vi "数据库配置.vi"() -> ()   [LabVIEW 2020]
uses:
  <vilib>/Utility/miscctls.llb/LVStringsAndValuesArrayTypeDef_U16.ctl
  <vilib>/addons/database/Connection.llb/DB Tools Open Connec (String).vi
  <vilib>/addons/database/Connection.llb/Conn Execute.vi
  <vilib>/addons/database/Recordset.llb/Rec Fetch Recordset Data (R).vi
  <vilib>/addons/database/Recordset.llb/Rec Destroy - Connection.vi
  <vilib>/addons/database/NI_Database_API.lvlib
panel:
  in  "取消":bool
  in  "确定":bool
  in  "数据库选择":enum32{"单机", "联机追溯"}(tab)
  out "数据库名称（单机）":string
  in  "使用文件名（单机）":string
  in  "打开路径（单机）":bool
  in  "数据库路径（单机）":string
  out "附加数据库（单机）":bool
  out "选择数据库（单机）":bool
  in  "在服务器上选择数据库（单机）":u16(ring) items=["CEPS", "D:\\LOCALDB.MDF", "SANLIserver"]
  in  "测试数据库（单机）":bool
  out "数据库信息":string
  in  "测试数据库（服务器）":bool
  in  "密码":string
  in  "用户名称":string
  in  "服务器名称（服务器）":string
  out "选择数据库（服务器）":bool
  in  "在服务器上选择数据库（服务器）":u16(ring)
  in  "使用文件名（服务器）":string
  in  "打开路径（服务器）":bool
  in  "数据库路径（服务器）":string
  out "附加数据库（服务器）":bool
  # "数据库名称"
  # "使用文件名"
  # "数据库信息"
  # "请输入登陆服务器信息："
  # "使用文件名"
  # "密码"
  # "用户名称"
  # "请输入服务器名称："
  # "服务器名称"
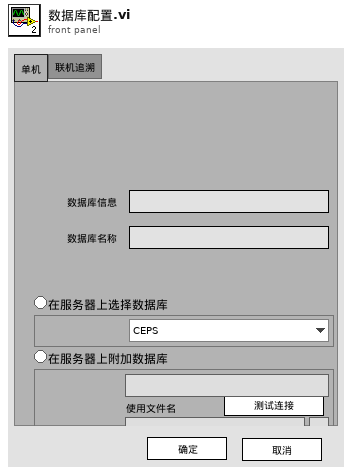
[diagram p1: front panel]
types:
  T1 = typedef "LVStringsAndValuesArrayTypeDef_U16.ctl" = cluster{"String":string, "Value":u16}[]
  T2 = enum8{"Enabled", "Disabled", "Disabled and Grayed Out"}
  T3 = typedef "NI_Database_API.lvlib/Conn ObjectReference.ctl" = refnum<k1>
  T4 = typedef "NI_Database_API.lvlib/Rec ObjectReference.ctl" = refnum<k1>
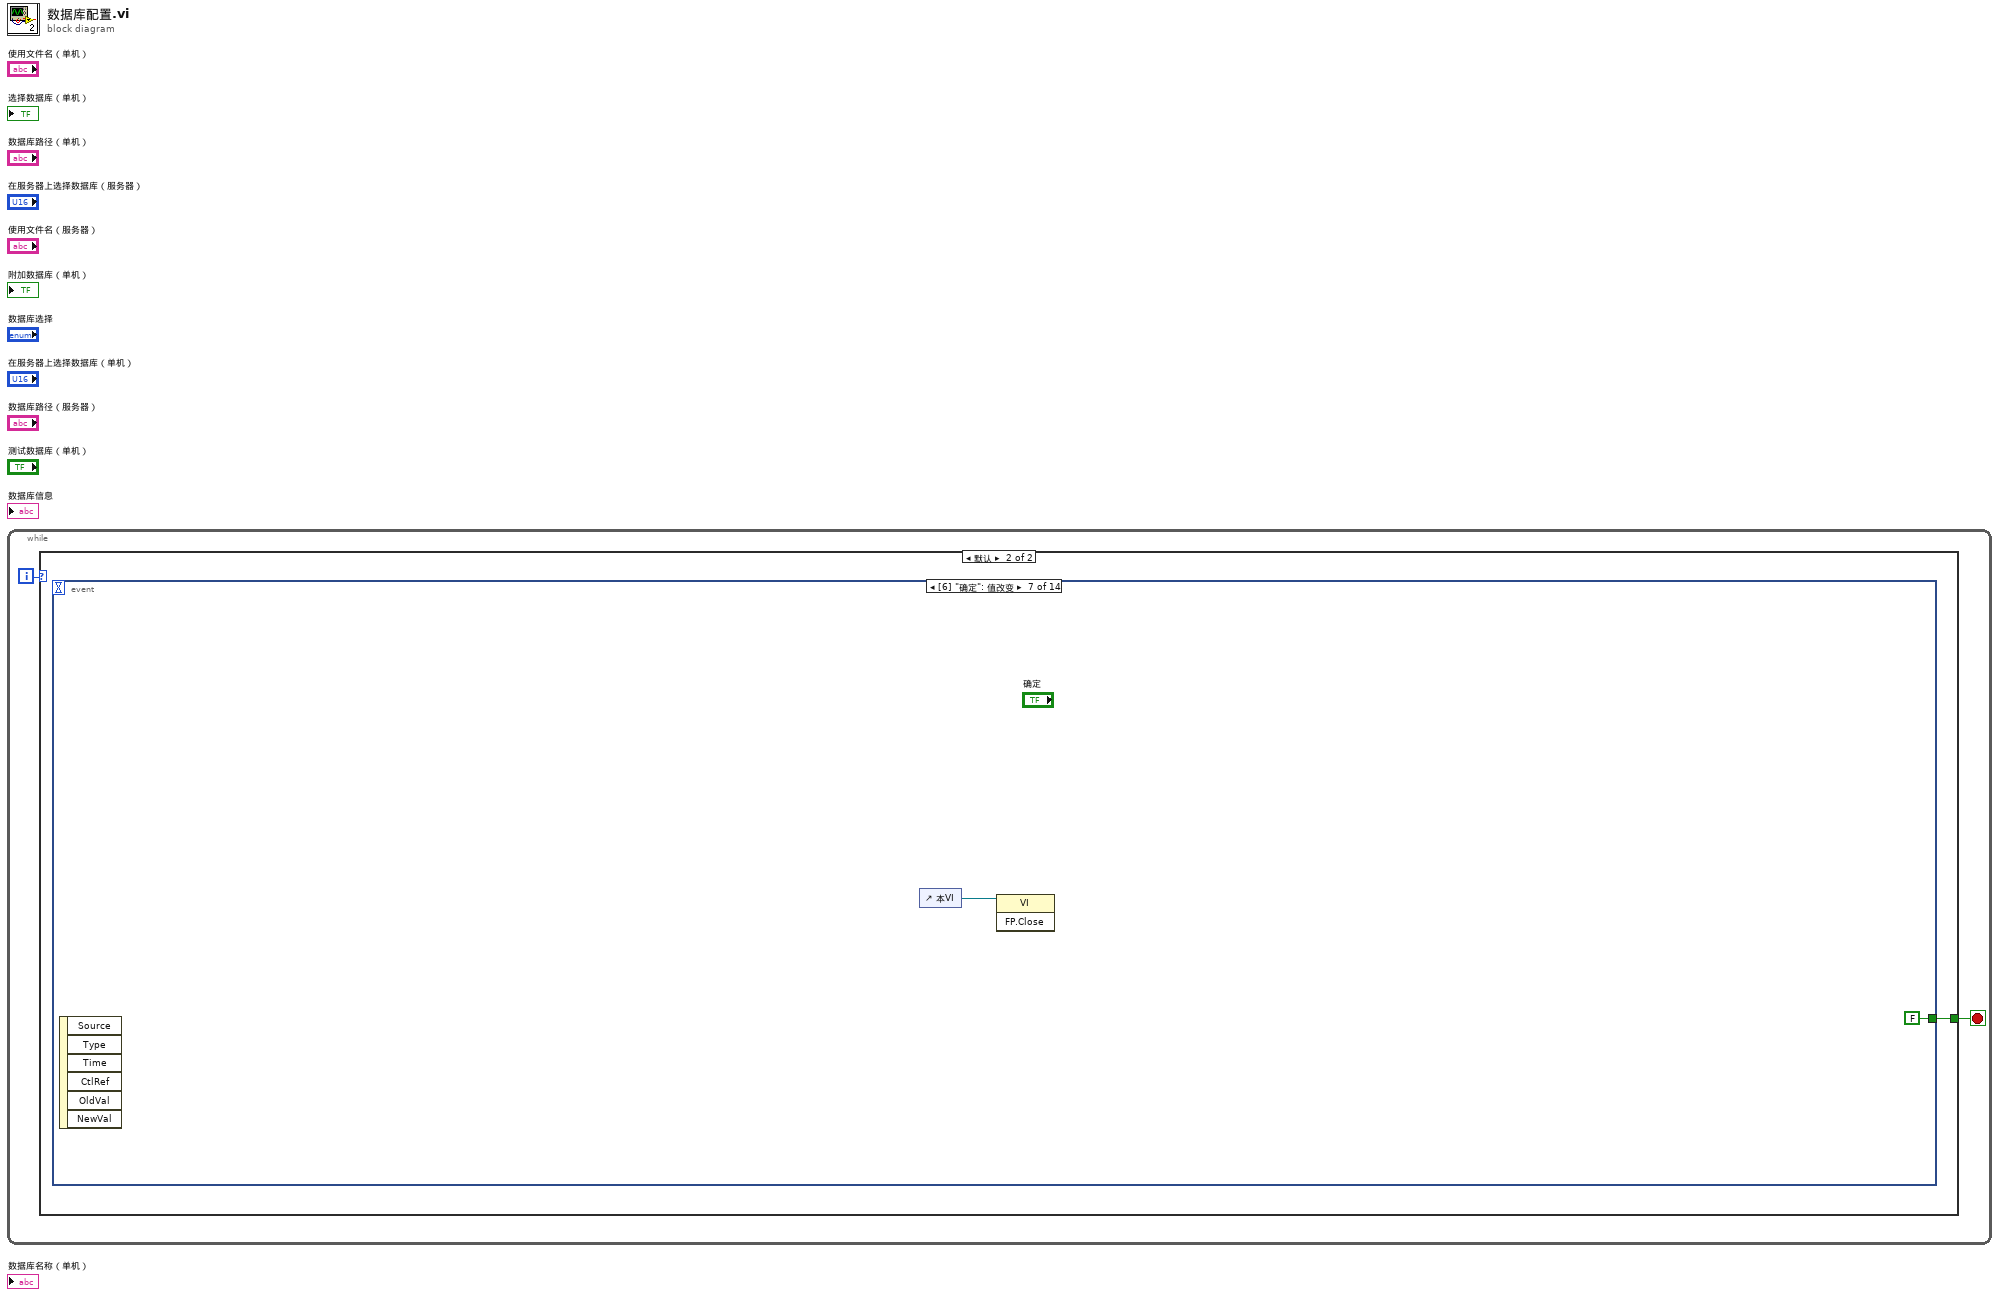
[diagram p0: block diagram]
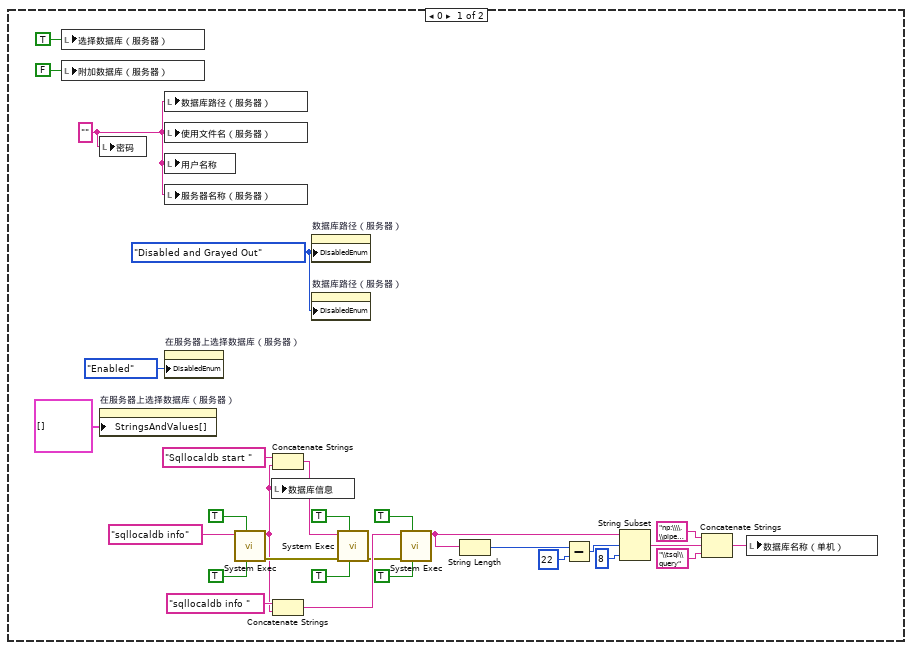
[diagram p2: hidden frame]
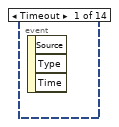
[diagram p3: hidden frame]
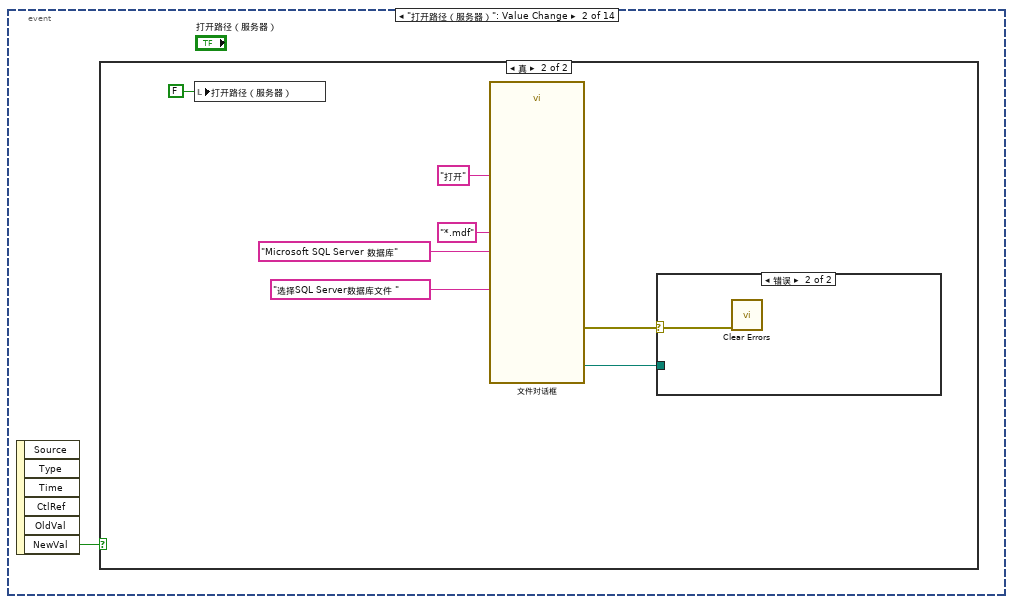
[diagram p4: hidden frame]
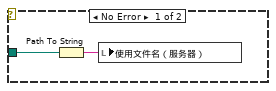
[diagram p6: hidden frame]
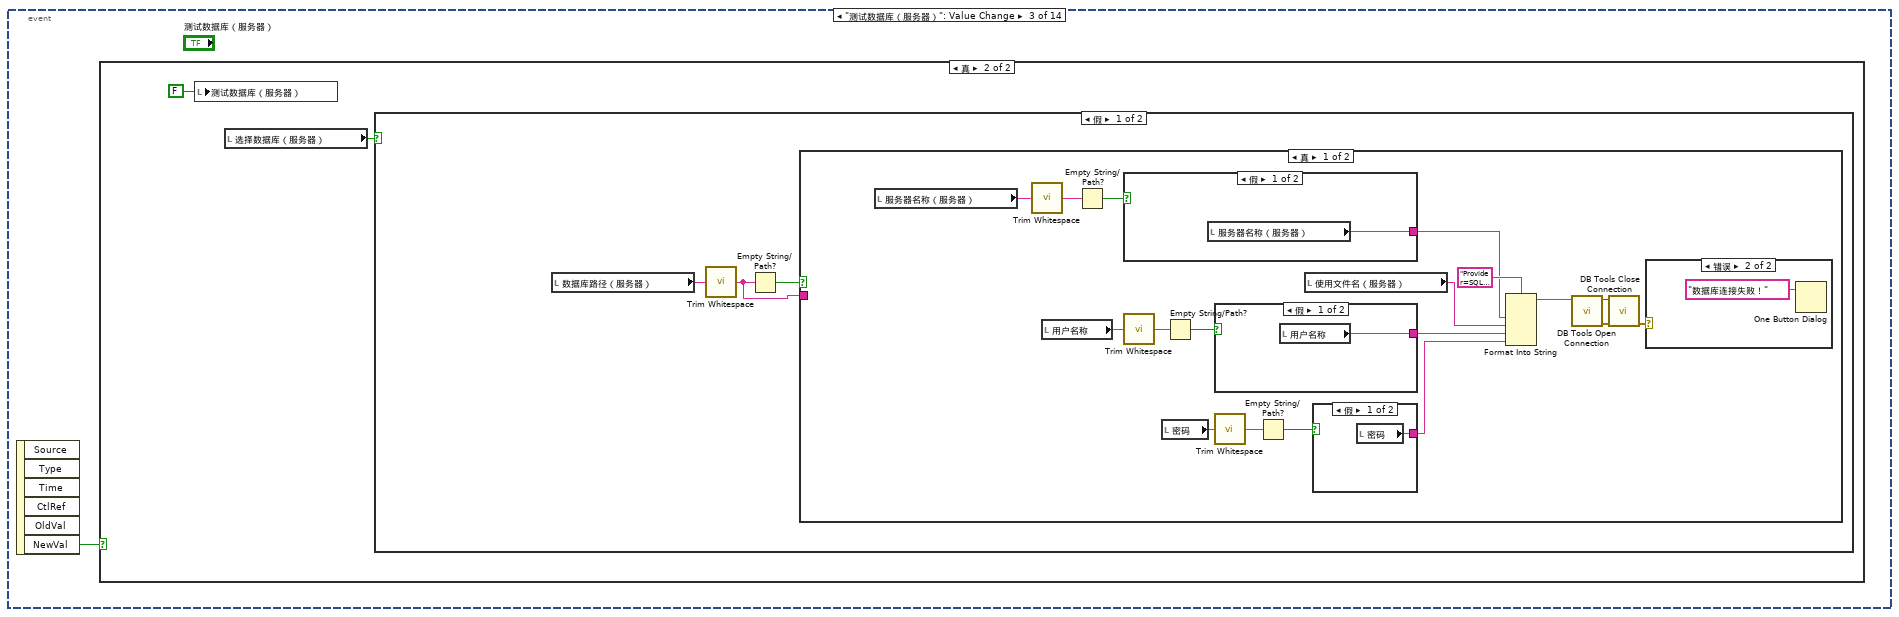
[diagram p7: hidden frame]
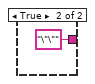
[diagram p9: hidden frame]
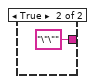
[diagram p10: hidden frame]
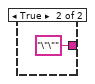
[diagram p11: hidden frame]
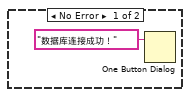
[diagram p12: hidden frame]
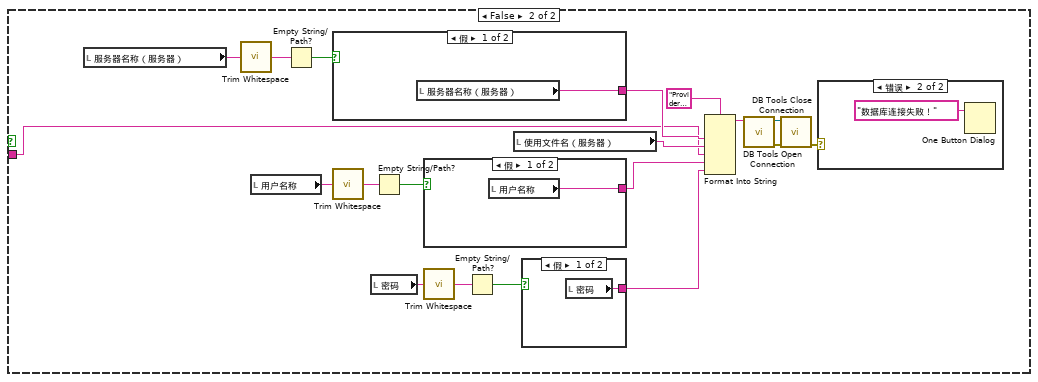
[diagram p13: hidden frame]
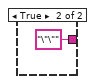
[diagram p14: hidden frame]
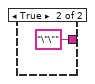
[diagram p15: hidden frame]
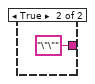
[diagram p16: hidden frame]
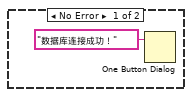
[diagram p17: hidden frame]
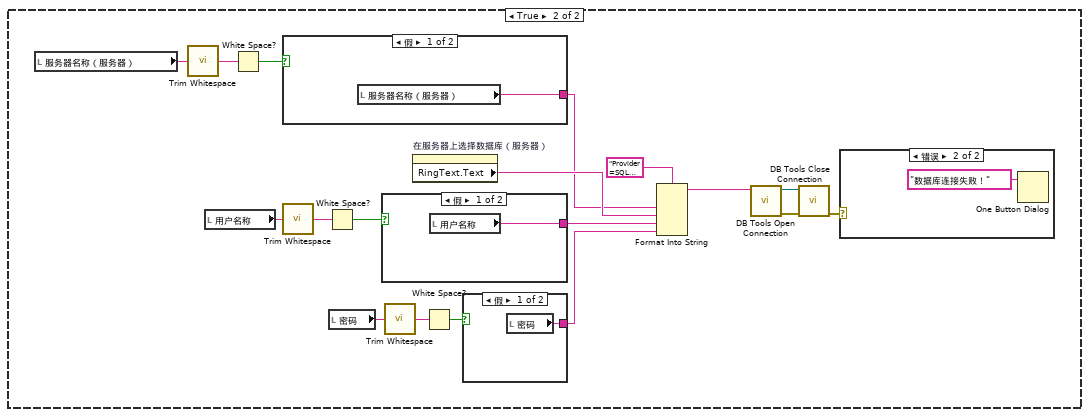
[diagram p18: hidden frame]
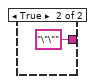
[diagram p19: hidden frame]
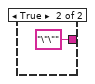
[diagram p20: hidden frame]
diagram:
  n1 = while {
    i -> [w1]
    stop <- w2 stop-if-true
    n2 = case shown="默认" w1 {
      tunnel: [_ w32] -> w2
      frame 0 {
        w27 = ""
        w31 = T2."Disabled and Grayed Out" ("禁用")
        n3 = local write "选择数据库（服务器）"(TRUE ("选择数据库（服务器）")) -> ()
        n4 = local write "附加数据库（服务器）"(FALSE ("附加数据库（服务器）")) -> ()
        n5 = local write "密码"(w27) -> ()
        n6 = property on="在服务器上选择数据库（服务器）" class="Ring (严格)"("StringsAndValues[]"=T1 [] ("字符串与值[]")) -> ()  [unwired: 2 in, 2 out]
        n7 = local write "数据库路径（服务器）"(w27) -> ()
        n8 = local write "使用文件名（服务器）"(w27) -> ()
        n9 = local write "用户名称"(w27) -> ()
        n10 = local write "服务器名称（服务器）"(w27) -> ()
        n11 = property on="在服务器上选择数据库（服务器）" class="Ring (严格)"("DisabledEnum"=T2."Enabled" ("禁用")) -> ()  [unwired: 2 in, 2 out]
        n12 = call <vilib>:"System Exec.vi"("run minimized? (F)"=TRUE, "wait until completion? (T)"=TRUE, "command line"="sqllocaldb info") -> ("error out"=w18:errorcluster, "standard output"=w5:string)  [unwired: 5 in, 2 out]
        n13 = local write "数据库信息"(w5) -> ()
        n14 = Concatenate Strings("Sqllocaldb start " ("command line"), w5) -> (w19:string)
        n15 = Concatenate Strings("sqllocaldb info " ("command line"), w5) -> (w17:string)
        n16 = property on="数据库路径（服务器）" class="Str"("DisabledEnum"=w31) -> ()  [unwired: 2 in, 2 out]
        n17 = property on="数据库路径（服务器）" class="Str"("DisabledEnum"=w31) -> ()  [unwired: 2 in, 2 out]
        n18 = call <vilib>:"System Exec.vi"("run minimized? (F)"=TRUE, "wait until completion? (T)"=TRUE, "error in (no error)"=w18, "command line"=w19) -> ("error out"=w4:errorcluster)  [unwired: 4 in, 3 out]
        n19 = call <vilib>:"System Exec.vi"("run minimized? (F)"=TRUE, "wait until completion? (T)"=TRUE, "error in (no error)"=w4, "command line"=w17) -> ("standard output"=w12:string)  [unwired: 4 in, 3 out]
        n20 = String Length(string=w12) -> (length=w13:i32)
        n21 = Subtract(x=w13, y=22) -> (x-y=w15:i32)
        n22 = String Subset(string=w12, offset (0)=w15, length (rest)=8 ("长度（剩余）")) -> (substring=w8:string)
        n23 = Concatenate Strings("np:\\\\.\\pipe\\LOCALDB#" ("格式字符串"), w8, "\\tsql\\query" ("字符串")) -> (w3:string)
        n24 = local write "数据库名称（单机）"(w3) -> ()
      }
      frame Default {
        n25 = event shown="[6] \"确定\": 值改变" {
          selector: _ -> [_ _ _ _ _ _ _ _ _ _ _ _ _ _]
          dyn-events: _ -> [_ _ _ _ _ _ _ _ _ _ _ _ _ _]
          timeout: _ -> [_ _ _ _ _ _ _ _ _ _ _ _ _ _]
          tunnel: [_ _ _ _ _ _ FALSE TRUE _ _ _ _ _ TRUE] -> w32
          event Timeout {
            n26 = event-data() -> ()  [unwired: 1 in, 3 out]
          }
          event "打开路径（服务器）": Value Change {
            n27 = event-data() -> ("NewVal"=w33:bool)  [unwired: 1 in, 5 out]
            n28 = case shown="真" w33 {
              frame False {
              }
              frame True {
                n29 = local write "打开路径（服务器）"(FALSE ("打开路径（服务器）")) -> ()
                n30 = call "文件对话框"("prompt"="选择SQL Server数据库文件 ", "button label"="打开", "pattern (all files)"="*.mdf", "pattern label"="Microsoft SQL Server 数据库") -> ("selected path"=w36:path, "error out"=w35:errorcluster)  [unwired: 8 in, 2 out]
                n31 = case shown="错误" w35 {
                  selector: w35 -> [_ w43]
                  tunnel: w36 -> [w42 _]
                  frame No Error {
                    n32 = Path To String(path=w42) -> (string=w41:string)
                    n33 = local write "使用文件名（服务器）"(w41) -> ()
                  }
                  frame Error {
                    n34 = call <vilib>:"Clear Errors.vi"("error in (no error)"=w43) -> ()  [unwired: 5 in, 2 out]
                  }
                }
              }
            }
          }
          event "测试数据库（服务器）": Value Change {
            n35 = event-data() -> ("NewVal"=w44:bool)  [unwired: 1 in, 5 out]
            n36 = case shown="真" w44 {
              frame False {
              }
              frame True {
                n37 = local write "测试数据库（服务器）"(FALSE ("测试数据库（服务器）")) -> ()
                n38 = local read "选择数据库（服务器）"() -> (w45:bool)
                n39 = case shown="假" w45 {
                  frame False {
                    n40 = local read "数据库路径（服务器）"() -> (w49:string)
                    n41 = call <vilib>:"Trim Whitespace.vi"("string"=w49) -> ("trimmed string"=w47:string)  [unwired: 1 in]
                    n42 = Empty String/Path?(string/path=w47) -> (empty?=w48:bool)
                    n43 = case shown="真" w48 {
                      tunnel: w47 -> [_ w76]
                      frame True {
                        n44 = local read "服务器名称（服务器）"() -> (w62:string)
                        n45 = call <vilib>:"Trim Whitespace.vi"("string"=w62) -> ("trimmed string"=w60:string)  [unwired: 1 in]
                        n46 = local read "用户名称"() -> (w57:string)
                        n47 = Empty String/Path?(string/path=w60) -> (empty?=w61:bool)
                        n48 = case shown="假" w61 {
                          tunnel: [w72 "\"\""] -> w59
                          frame False {
                            n49 = local read "服务器名称（服务器）"() -> (w72:string)
                          }
                          frame True {
                          }
                        }
                        n50 = call <vilib>:"Trim Whitespace.vi"("string"=w57) -> ("trimmed string"=w53:string)  [unwired: 1 in]
                        n51 = local read "密码"() -> (w58:string)
                        n52 = Empty String/Path?(string/path=w53) -> (empty?=w54:bool)
                        n53 = case shown="假" w54 {
                          tunnel: [w70 "\"\""] -> w52
                          frame False {
                            n54 = local read "用户名称"() -> (w70:string)
                          }
                          frame True {
                          }
                        }
                        n55 = call <vilib>:"Trim Whitespace.vi"("string"=w58) -> ("trimmed string"=w55:string)  [unwired: 1 in]
                        n56 = Empty String/Path?(string/path=w55) -> (empty?=w56:bool)
                        n57 = local read "使用文件名（服务器）"() -> (w50:string)
                        n58 = case shown="假" w56 {
                          tunnel: [w68 "\"\""] -> w51
                          frame False {
                            n59 = local read "密码"() -> (w68:string)
                          }
                          frame True {
                          }
                        }
                        n60 = Format Into String(format string="Provider=SQLOLEDB.1;Integrated Security=SSPI;Persist Security Info=True;Data Source=%s;Initial File Name=%s;User ID=%s;Password=%s" ("格式字符串"), w59, w50, w52, w51) -> (resulting string=w65:string)  [unwired: 2 in, 1 out]
                        n61 = call-poly <vilib>:"DB Tools Open Connection.vi"("connection information"=w65) -> ("error out"=w66:errorcluster, "connection reference"=w67:T3)  [unwired: 7 in]
                        n62 = call <vilib>:"DB Tools Close Connection.vi"("error in (no error)"=w66, "connection reference"=w67) -> ("error out"=w64:errorcluster)  [unwired: 5 in]
                        n63 = case shown="错误" w64 {
                          frame No Error {
                            n64 = One Button Dialog(message="数据库连接成功！" ("消息")) -> ()  [unwired: 1 in, 1 out]
                          }
                          frame Error {
                            n65 = One Button Dialog(message="数据库连接失败！" ("消息")) -> ()  [unwired: 1 in, 1 out]
                          }
                        }
                      }
                      frame False {
                        n66 = local read "服务器名称（服务器）"() -> (w89:string)
                        n67 = call <vilib>:"Trim Whitespace.vi"("string"=w89) -> ("trimmed string"=w87:string)  [unwired: 1 in]
                        n68 = local read "用户名称"() -> (w84:string)
                        n69 = Empty String/Path?(string/path=w87) -> (empty?=w88:bool)
                        n70 = case shown="假" w88 {
                          tunnel: [w99 "\"\""] -> w86
                          frame False {
                            n71 = local read "服务器名称（服务器）"() -> (w99:string)
                          }
                          frame True {
                          }
                        }
                        n72 = call <vilib>:"Trim Whitespace.vi"("string"=w84) -> ("trimmed string"=w80:string)  [unwired: 1 in]
                        n73 = local read "密码"() -> (w85:string)
                        n74 = Empty String/Path?(string/path=w80) -> (empty?=w81:bool)
                        n75 = case shown="假" w81 {
                          tunnel: [w97 "\"\""] -> w77
                          frame False {
                            n76 = local read "用户名称"() -> (w97:string)
                          }
                          frame True {
                          }
                        }
                        n77 = call <vilib>:"Trim Whitespace.vi"("string"=w85) -> ("trimmed string"=w82:string)  [unwired: 1 in]
                        n78 = Empty String/Path?(string/path=w82) -> (empty?=w83:bool)
                        n79 = local read "使用文件名（服务器）"() -> (w79:string)
                        n80 = case shown="假" w83 {
                          tunnel: [w95 "\"\""] -> w78
                          frame False {
                            n81 = local read "密码"() -> (w95:string)
                          }
                          frame True {
                          }
                        }
                        n82 = Format Into String(format string="Provider=SQLOLEDB.1;Integrated Security=SSPI;Persist Security Info=True;Data Source=%s;Initial File Name=%s;Initial Catalog=%s;User ID=%s;Password=%s" ("格式字符串"), w86, w79, w76, w77, w78) -> (resulting string=w92:string)  [unwired: 2 in, 1 out]
                        n83 = call-poly <vilib>:"DB Tools Open Connection.vi"("connection information"=w92) -> ("error out"=w93:errorcluster, "connection reference"=w94:T3)  [unwired: 7 in]
                        n84 = call <vilib>:"DB Tools Close Connection.vi"("error in (no error)"=w93, "connection reference"=w94) -> ("error out"=w91:errorcluster)  [unwired: 5 in]
                        n85 = case shown="错误" w91 {
                          frame No Error {
                            n86 = One Button Dialog(message="数据库连接成功！" ("消息")) -> ()  [unwired: 1 in, 1 out]
                          }
                          frame Error {
                            n87 = One Button Dialog(message="数据库连接失败！" ("消息")) -> ()  [unwired: 1 in, 1 out]
                          }
                        }
                      }
                    }
                  }
                  frame True {
                    n88 = local read "服务器名称（服务器）"() -> (w114:string)
                    n89 = call <vilib>:"Trim Whitespace.vi"("string"=w114) -> ("trimmed string"=w112:string)  [unwired: 1 in]
                    n90 = local read "用户名称"() -> (w109:string)
                    n91 = White Space?(1:w112) -> (0:w113:bool)
                    n92 = case shown="假" w113 {
                      tunnel: [w125 "\"\""] -> w111
                      frame False {
                        n93 = local read "服务器名称（服务器）"() -> (w125:string)
                      }
                      frame True {
                      }
                    }
                    n94 = call <vilib>:"Trim Whitespace.vi"("string"=w109) -> ("trimmed string"=w105:string)  [unwired: 1 in]
                    n95 = White Space?(1:w105) -> (0:w106:bool)
                    n96 = local read "密码"() -> (w110:string)
                    n97 = case shown="假" w106 {
                      tunnel: [w123 "\"\""] -> w104
                      frame False {
                        n98 = local read "用户名称"() -> (w123:string)
                      }
                      frame True {
                      }
                    }
                    n99 = call <vilib>:"Trim Whitespace.vi"("string"=w110) -> ("trimmed string"=w107:string)  [unwired: 1 in]
                    n100 = property on="在服务器上选择数据库（服务器）" class="Ring (严格)"() -> ("RingText.Text"=w117:string)  [unwired: 2 in, 2 out]
                    n101 = White Space?(1:w107) -> (0:w108:bool)
                    n102 = case shown="假" w108 {
                      tunnel: [w121 "\"\""] -> w103
                      frame False {
                        n103 = local read "密码"() -> (w121:string)
                      }
                      frame True {
                      }
                    }
                    n104 = Format Into String(format string="Provider=SQLOLEDB.1;Integrated Security=SSPI;Persist Security Info=True;Data Source=%s;Initial Catalog=%s;User ID=%s;Password=%s" ("格式字符串"), w111, w117, w104, w103) -> (resulting string=w118:string)  [unwired: 2 in, 1 out]
                    n105 = call-poly <vilib>:"DB Tools Open Connection.vi"("connection information"=w118) -> ("error out"=w119:errorcluster, "connection reference"=w120:T3)  [unwired: 7 in]
                    n106 = call <vilib>:"DB Tools Close Connection.vi"("error in (no error)"=w119, "connection reference"=w120) -> ("error out"=w116:errorcluster)  [unwired: 5 in]
                    n107 = case shown="错误" w116 {
                      frame No Error {
                        n108 = One Button Dialog(message="数据库连接成功！" ("消息")) -> ()  [unwired: 1 in, 1 out]
                      }
                      frame Error {
                        n109 = One Button Dialog(message="数据库连接失败！" ("消息")) -> ()  [unwired: 1 in, 1 out]
                      }
                    }
                  }
                }
              }
            }
          }
          event "选择数据库（服务器）": Mouse Down {
            w129 = ""
            w130 = T2."Disabled and Grayed Out" ("禁用")
            n110 = event-data() -> ()  [unwired: 1 in, 8 out]
            n111 = local write "附加数据库（服务器）"(FALSE ("附加数据库（服务器）")) -> ()
            n112 = local write "选择数据库（服务器）"(TRUE ("选择数据库（服务器）")) -> ()
            n113 = local write "使用文件名（服务器）"(w129) -> ()
            n114 = local write "数据库路径（服务器）"(w129) -> ()
            n115 = property on="在服务器上选择数据库（服务器）" class="Ring (严格)"("DisabledEnum"=T2."Enabled" ("禁用")) -> ()  [unwired: 2 in, 2 out]
            n116 = property on="数据库路径（服务器）" class="Str"("DisabledEnum"=w130) -> ()  [unwired: 2 in, 2 out]
            n117 = property on="打开路径（服务器）" class="Bool (严格)"("DisabledEnum"=w130) -> ()  [unwired: 2 in, 2 out]
            n118 = property on="使用文件名（服务器）" class="Str"("DisabledEnum"=w130) -> ()  [unwired: 2 in, 2 out]
          }
          event "附加数据库（服务器）": Mouse Down {
            w135 = T2."Enabled" ("禁用")
            n119 = event-data() -> ()  [unwired: 1 in, 8 out]
            n120 = local write "选择数据库（服务器）"(FALSE ("选择数据库（服务器）")) -> ()
            n121 = local write "附加数据库（服务器）"(TRUE ("附加数据库（服务器）")) -> ()
            n122 = property on="在服务器上选择数据库（服务器）" class="Ring (严格)"("StringsAndValues[]"=T1 [] ("字符串与值[]")) -> ()  [unwired: 2 in, 2 out]
            n123 = property on="数据库路径（服务器）" class="Str"("DisabledEnum"=w135) -> ()  [unwired: 2 in, 2 out]
            n124 = property on="打开路径（服务器）" class="Bool (严格)"("DisabledEnum"=w135) -> ()  [unwired: 2 in, 2 out]
            n125 = property on="使用文件名（服务器）" class="Str"("DisabledEnum"=w135) -> ()  [unwired: 2 in, 2 out]
            n126 = property on="在服务器上选择数据库（服务器）" class="Ring (严格)"("DisabledEnum"=T2."Disabled and Grayed Out" ("禁用")) -> ()  [unwired: 2 in, 2 out]
          }
          event "在服务器上选择数据库（服务器）": Mouse Down {
            n127 = event-data() -> ()  [unwired: 1 in, 8 out]
            n128 = call <vilib>:"Trim Whitespace.vi"("string"="服务器名称（服务器）") -> ("trimmed string"=w141:string)  [unwired: 1 in]
            n129 = Empty String/Path?(string/path=w141) -> (empty?=w146:bool)
            n130 = case shown="假" w146 {
              tunnel: [w168 "\"\""] -> w144
              frame False {
                n131 = local read "服务器名称（服务器）"() -> (w168:string)
              }
              frame True {
              }
            }
            n132 = call <vilib>:"Trim Whitespace.vi"("string"="用户名称") -> ("trimmed string"=w140:string)  [unwired: 1 in]
            n133 = Empty String/Path?(string/path=w140) -> (empty?=w147:bool)
            n134 = case shown="真" w147 {
              tunnel: [w172 "\"\""] -> w143
              frame False {
                n135 = local read "用户名称"() -> (w172:string)
              }
              frame True {
              }
            }
            n136 = call <vilib>:"Trim Whitespace.vi"("string"="密码") -> ("trimmed string"=w139:string)  [unwired: 1 in]
            n137 = Empty String/Path?(string/path=w139) -> (empty?=w145:bool)
            n138 = case shown="真" w145 {
              tunnel: [w170 "\"\""] -> w142
              frame False {
                n139 = local read "密码"() -> (w170:string)
              }
              frame True {
              }
            }
            n140 = Format Into String(format string="Provider=SQLOLEDB.1;Integrated Security=SSPI;Persist Security Info=False;Data Source=%s;User ID=%s;Password=%s" ("格式字符串"), w144, w143, w142) -> (resulting string=w164:string, error out=w149:errorcluster)  [unwired: 2 in]
            n141 = call-poly <vilib>:"DB Tools Open Connection.vi"("error in (no error)"=w149, "connection information"=w164) -> ("error out"=w154:errorcluster, "connection reference"=w163:T3)  [unwired: 6 in]
            n142 = call-poly <vilib>:"DB Tools Execute Query.vi"("error in (no error)"=w154, "SQL query"="SELECT Name FROM Master..SysDatabases where dbid>4 ORDER BY Name", "connection reference"=w163) -> ("error out"=w161:errorcluster, "recordset reference"=w160:T4)  [unwired: 5 in]
            n143 = call-poly <vilib>:"DB Tools Fetch Recordset Data.vi"("error in (no error)"=w161, "recordset reference"=w160) -> ("error out"=w152:errorcluster, "recordset data"=w159:variant[][], "recordset reference out"=w153:T4)  [unwired: 3 in]
            n144 = call-poly <vilib>:"DB Tools Free Object.vi"("error in (no error)"=w152, "recordset reference"=w153) -> ("error out"=w151:errorcluster, "connection reference"=w150:T3)  [unwired: 8 in]
            n145 = Variant To Data(type=string[][] [] ("字符串[]"), Variant=w159) -> (data=w157:string[][])  [unwired: 1 in, 1 out]
            n146 = call <vilib>:"DB Tools Close Connection.vi"("error in (no error)"=w151, "connection reference"=w150) -> ()  [unwired: 5 in, 1 out]
            n147 = Index Array(array=w157, index (col)=0 ("禁用的索引 (列)")) -> (element=w156:string[])  [unwired: 1 in]
            n148 = property on="在服务器上选择数据库（服务器）" class="Ring (严格)"("Strings []"=w156) -> ()  [unwired: 2 in, 2 out]
          }
          event "确定": Value Change {
            n149 = event-data() -> ()  [unwired: 1 in, 6 out]
            n150 = control-ref of="本VI"() -> (w174:refnum<vi>)
            n151 = invoke class="VI" method="FP.Close"(reference=w174) -> ()  [unwired: 2 in, 3 out]
          }
          event "取消": Value Change {
            n152 = event-data() -> ()  [unwired: 1 in, 6 out]
            n153 = control-ref of="本VI"() -> (w176:refnum<vi>)
            n154 = invoke class="VI" method="FP.Close"(reference=w176) -> ()  [unwired: 2 in, 3 out]
          }
          event "选择数据库（单机）": Mouse Down {
            w180 = "" ("使用文件名（单机）")
            w178 = T2."Disabled and Grayed Out" ("禁用")
            n155 = event-data() -> ()  [unwired: 1 in, 8 out]
            n156 = local write "附加数据库（单机）"(FALSE ("附加数据库（单机）")) -> ()
            n157 = local write "选择数据库（单机）"(TRUE ("选择数据库（单机）")) -> ()
            n158 = local write "使用文件名（单机）"(w180) -> ()
            n159 = local write "数据库路径（单机）"(w180) -> ()
            n160 = property on="在服务器上选择数据库（单机）" class="Ring (严格)"("DisabledEnum"=T2."Enabled" ("禁用")) -> ()  [unwired: 2 in, 2 out]
            n161 = property on="打开路径（单机）" class="Bool (严格)"("DisabledEnum"=w178) -> ()  [unwired: 2 in, 2 out]
            n162 = property on="数据库路径（单机）" class="Str"("DisabledEnum"=w178) -> ()  [unwired: 2 in, 2 out]
            n163 = property on="使用文件名（单机）" class="Str"("DisabledEnum"=w178) -> ()  [unwired: 2 in, 2 out]
          }
          event "附加数据库（单机）": Mouse Down {
            w187 = T2."Enabled" ("禁用")
            n164 = event-data() -> ()  [unwired: 1 in, 8 out]
            n165 = local write "选择数据库（单机）"(FALSE ("选择数据库（单机）")) -> ()
            n166 = local write "附加数据库（单机）"(TRUE ("附加数据库（单机）")) -> ()
            n167 = property on="在服务器上选择数据库（单机）" class="Ring (严格)"("StringsAndValues[]"=T1 [] ("字符串与值[]")) -> ()  [unwired: 2 in, 2 out]
            n168 = property on="使用文件名（单机）" class="Str"("DisabledEnum"=w187) -> ()  [unwired: 2 in, 2 out]
            n169 = property on="数据库路径（单机）" class="Str"("DisabledEnum"=w187) -> ()  [unwired: 2 in, 2 out]
            n170 = property on="打开路径（单机）" class="Bool (严格)"("DisabledEnum"=w187) -> ()  [unwired: 2 in, 2 out]
            n171 = property on="在服务器上选择数据库（单机）" class="Ring (严格)"("DisabledEnum"=T2."Disabled and Grayed Out" ("禁用")) -> ()  [unwired: 2 in, 2 out]
          }
          event "测试数据库（单机）": Value Change {
            n172 = event-data() -> ("NewVal"=w188:bool)  [unwired: 1 in, 5 out]
            n173 = case shown="真" w188 {
              frame False {
              }
              frame True {
                n174 = local write "测试数据库（单机）"(FALSE ("测试数据库（单机）")) -> ()
                n175 = local read "选择数据库（单机）"() -> (w189:bool)
                n176 = case shown="假" w189 {
                  frame False {
                    n177 = local read "数据库路径（单机）"() -> (w191:string)
                    n178 = White Space?(1:w191) -> (0:w192:bool)
                    n179 = case shown="假" w192 {
                      tunnel: w191 -> [_ w203]
                      frame True {
                        n180 = local read "使用文件名（单机）"() -> (w193:string)
                        n181 = local read "数据库名称（单机）"() -> (w194:string)
                        n182 = Format Into String(format string="Provider=SQLOLEDB.1;Integrated Security=SSPI;Persist Security Info=True;Initial File Name=%s;Data Source=" ("格式字符串"), w193) -> (resulting string=w197:string)  [unwired: 2 in, 1 out]
                        n183 = Concatenate Strings(w197, w194) -> (w196:string)
                        n184 = call-poly <vilib>:"DB Tools Open Connection.vi"("connection information"=w196) -> ("error out"=w199:errorcluster, "connection reference"=w200:T3)  [unwired: 7 in]
                        n185 = call <vilib>:"DB Tools Close Connection.vi"("error in (no error)"=w199, "connection reference"=w200) -> ("error out"=w198:errorcluster)  [unwired: 5 in]
                        n186 = case shown="错误" w198 {
                          frame No Error {
                            n187 = One Button Dialog(message="数据库连接成功！" ("消息")) -> ()  [unwired: 1 in, 1 out]
                          }
                          frame Error {
                            n188 = One Button Dialog(message="数据库连接失败！" ("消息")) -> ()  [unwired: 1 in, 1 out]
                          }
                        }
                      }
                      frame False {
                        n189 = local read "使用文件名（单机）"() -> (w205:string)
                        n190 = local read "数据库名称（单机）"() -> (w204:string)
                        n191 = Format Into String(format string="Provider=SQLOLEDB.1;Integrated Security=SSPI;Persist Security Info=True;Initial File Name=%s;Initial Catalog=%s;Data Source=" ("格式字符串"), w205, w203) -> (resulting string=w208:string)  [unwired: 2 in, 1 out]
                        n192 = Concatenate Strings(w208, w204) -> (w207:string)
                        n193 = call-poly <vilib>:"DB Tools Open Connection.vi"("connection information"=w207) -> ("error out"=w210:errorcluster, "connection reference"=w211:T3)  [unwired: 7 in]
                        n194 = call <vilib>:"DB Tools Close Connection.vi"("error in (no error)"=w210, "connection reference"=w211) -> ("error out"=w209:errorcluster)  [unwired: 5 in]
                        n195 = case shown="错误" w209 {
                          frame No Error {
                            n196 = One Button Dialog(message="数据库连接成功！" ("消息")) -> ()  [unwired: 1 in, 1 out]
                          }
                          frame Error {
                            n197 = One Button Dialog(message="数据库连接失败！" ("消息")) -> ()  [unwired: 1 in, 1 out]
                          }
                        }
                      }
                    }
                  }
                  frame True {
                    n198 = property on="在服务器上选择数据库（单机）" class="Ring (严格)"() -> ("RingText.Text"=w218:string)  [unwired: 2 in, 2 out]
                    n199 = local read "数据库名称（单机）"() -> (w214:string)
                    n200 = Format Into String(format string="Provider=SQLOLEDB.1;Integrated Security=SSPI;Persist Security Info=True;Initial Catalog=%s;Data Source=" ("格式字符串"), w218) -> (resulting string=w217:string)  [unwired: 2 in, 1 out]
                    n201 = Concatenate Strings(w217, w214) -> (w216:string)
                    n202 = call-poly <vilib>:"DB Tools Open Connection.vi"("connection information"=w216) -> ("error out"=w220:errorcluster, "connection reference"=w221:T3)  [unwired: 7 in]
                    n203 = call <vilib>:"DB Tools Close Connection.vi"("error in (no error)"=w220, "connection reference"=w221) -> ("error out"=w219:errorcluster)  [unwired: 5 in]
                    n204 = case shown="错误" w219 {
                      frame No Error {
                        n205 = One Button Dialog(message="数据库连接成功！" ("消息")) -> ()  [unwired: 1 in, 1 out]
                      }
                      frame Error {
                        n206 = One Button Dialog(message="数据库连接失败！" ("消息")) -> ()  [unwired: 1 in, 1 out]
                      }
                    }
                  }
                }
              }
            }
          }
          event "在服务器上选择数据库（单机）": Mouse Down {
            n207 = event-data() -> ()  [unwired: 1 in, 8 out]
            n208 = local read "数据库名称（单机）"() -> (w224:string)
            n209 = Concatenate Strings("Provider=SQLOLEDB.1;Integrated Security=SSPI;Persist Security Info=False;Data Source=" ("格式字符串"), w224) -> (w225:string)
            n210 = call-poly <vilib>:"DB Tools Open Connection.vi"("connection information"=w225) -> ("error out"=w233:errorcluster, "connection reference"=w240:T3)  [unwired: 7 in]
            n211 = call-poly <vilib>:"DB Tools Execute Query.vi"("error in (no error)"=w233, "SQL query"="SELECT Name FROM Master..SysDatabases where dbid>4 ORDER BY Name", "connection reference"=w240) -> ("error out"=w238:errorcluster, "recordset reference"=w237:T4)  [unwired: 5 in]
            n212 = call-poly <vilib>:"DB Tools Fetch Recordset Data.vi"("error in (no error)"=w238, "recordset reference"=w237) -> ("error out"=w231:errorcluster, "recordset data"=w236:variant[][], "recordset reference out"=w232:T4)  [unwired: 3 in]
            n213 = call-poly <vilib>:"DB Tools Free Object.vi"("error in (no error)"=w231, "recordset reference"=w232) -> ("error out"=w230:errorcluster, "connection reference"=w229:T3)  [unwired: 8 in]
            n214 = Variant To Data(type=string[][] [] ("字符串[]"), Variant=w236) -> (data=w235:string[][])  [unwired: 1 in, 1 out]
            n215 = call <vilib>:"DB Tools Close Connection.vi"("error in (no error)"=w230, "connection reference"=w229) -> ()  [unwired: 5 in, 1 out]
            n216 = Index Array(array=w235, index (col)=0 ("禁用的索引 (列)")) -> (element=w227:string[])  [unwired: 1 in]
            n217 = property on="在服务器上选择数据库（单机）" class="Ring (严格)"("Strings []"=w227) -> ()  [unwired: 2 in, 2 out]
          }
          event "打开路径（单机）": Value Change {
            n218 = event-data() -> ("NewVal"=w241:bool)  [unwired: 1 in, 5 out]
            n219 = case shown="真" w241 {
              frame False {
              }
              frame True {
                n220 = local write "打开路径（单机）"(FALSE ("打开路径（单机）")) -> ()
                n221 = call "文件对话框"("prompt"="选择SQL Server数据库文件 ", "button label"="打开", "pattern (all files)"="*.mdf", "pattern label"="Microsoft SQL Server 数据库") -> ("selected path"=w244:path, "error out"=w243:errorcluster)  [unwired: 8 in, 2 out]
                n222 = case shown="错误" w243 {
                  selector: w243 -> [_ w251]
                  tunnel: w244 -> [w250 _]
                  frame No Error {
                    n223 = Path To String(path=w250) -> (string=w249:string)
                    n224 = local write "使用文件名（单机）"(w249) -> ()
                  }
                  frame Error {
                    n225 = call <vilib>:"Clear Errors.vi"("error in (no error)"=w251) -> ()  [unwired: 5 in, 2 out]
                  }
                }
              }
            }
          }
          event Panel Close {
            n226 = event-data() -> ()  [unwired: 1 in, 4 out]
          }
        }
      }
    }
  }
